vi "GoToAbsPos.vi"(0 "object in":refnum<class "Prior_Zmotor.lvclass">, 2 "Pos (um)":i32, 5 "error in (no error)":errorcluster) -> (14 "object out":refnum<class "Prior_Zmotor.lvclass">, 16 "read buffer":string, 19 "error out":errorcluster)   [LabVIEW 2021, in "Prior_Zmotor.lvclass"]
uses:
  Prior_Zmotor.lvclass
  Prior_Zmotor.lvclass/Prior_Zmotor.ctl
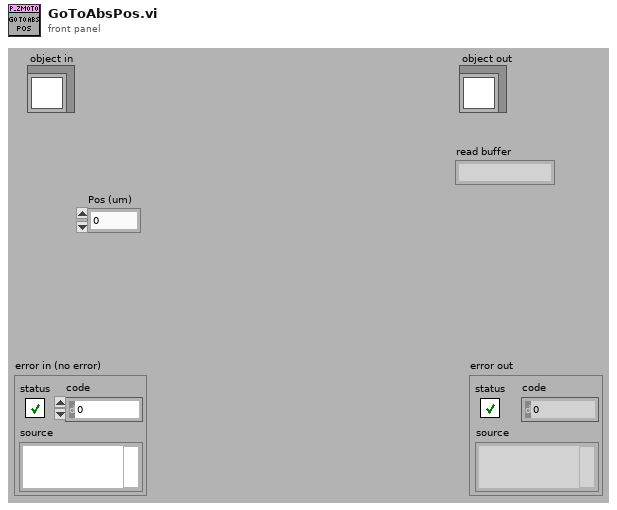
[diagram p1: front panel]
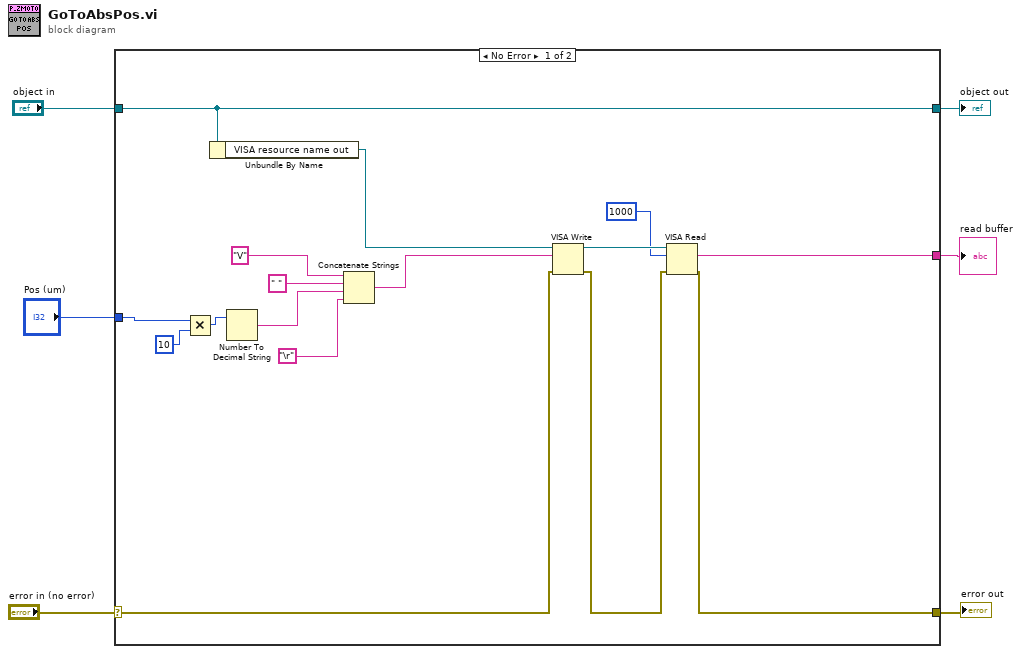
[diagram p0: block diagram]
diagram:
  n1 = case shown="No Error" "error in (no error)" {
    selector: "error in (no error)" -> [w20 w24]
    tunnel: [w12 w24] -> w5
    tunnel: [w22 w23] -> w3
    tunnel: "object in" -> [w22 w23]
    tunnel: "Pos (um)" -> [w16 _]
    tunnel: [w10 _] -> w1
    frame No Error {
      n2 = Multiply(x=w16, y=10) -> (x*y=w17:i32)
      n3 = Unbundle By Name(w22) -> ("VISA resource name out"=w21:refnum<visa-resource-name>)
      n4 = Number To Decimal String(number=w17) -> (decimal integer string=w19:string)  [unwired: 1 in]
      n5 = Concatenate Strings("V" ("write buffer"), " " ("string"), w19, "\r") -> (w7:string)
      n6 = VISA Write(VISA resource name=w21, write buffer=w7, error in (no error)=w20) -> (VISA resource name out=w14:refnum<visa-resource-name>, error out=w13:errorcluster)  [unwired: 1 out]
      n7 = VISA Read(VISA resource name=w14, byte count=u32 1000, error in (no error)=w13) -> (read buffer=w10:string, error out=w12:errorcluster)  [unwired: 2 out]
    }
    frame Error {
    }
  }
  "error out" <- w5
  "object out" <- w3
  "read buffer" <- w1
